vi "LCR_Readout.vi"(8 "error in (no error)":errorcluster, 11 "HP4284A in":refnum<class "HP4284A.lvclass">) -> (0 "error out":errorcluster, 1 "Resistance in Ohm":dbl, 2 "Capacitance in pF":dbl, 3 "HP4284A out":refnum<class "HP4284A.lvclass">)   [LabVIEW 2018, in "HP4284A.lvclass"]
uses:
  HP4284A.lvclass
panel:
  out "Data status":i32
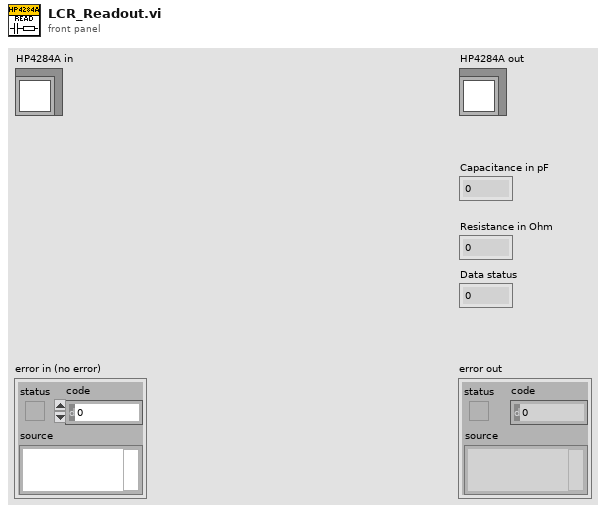
[diagram p1: front panel]
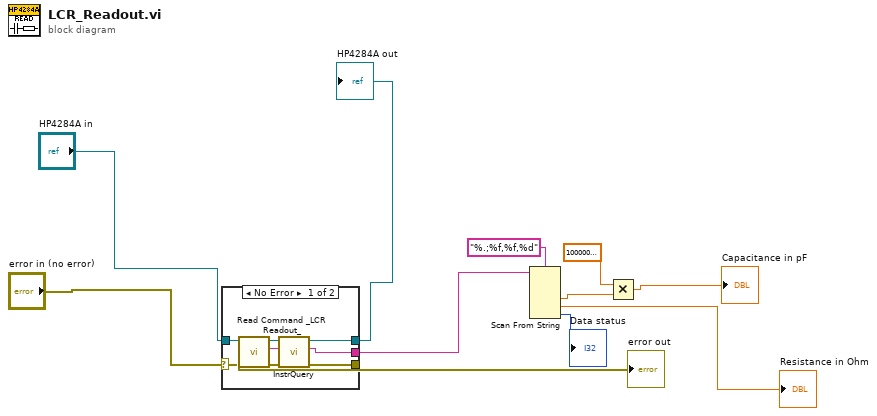
[diagram p0: block diagram]
diagram:
  n1 = case shown="No Error" "error in (no error)" {
    selector: "error in (no error)" -> [w15 w21]
    tunnel: [w14 w21] -> w11
    tunnel: [w19 w20] -> w10
    tunnel: "HP4284A in" -> [w13 w20]
    tunnel: [w12 _] -> w6
    frame No Error {
      n2 = call-dynamic "Read Command _LCR Readout_.vi"("error in (no error)"=w15, "LCRControl in"=w13) -> ("error out"=w16:errorcluster, "Command \"LCR Readout\""=w17:string, "LCRControl out"=w18:refnum<class "HP4284A.lvclass">)  [unwired: 7 in]
      n3 = call-dynamic "InstrQuery.vi"("error in (no error)"=w16, "Command string"=w17, "InstControl in"=w18) -> ("error out"=w14:errorcluster, "Instrument response"=w12:string, "InstControl out"=w19:refnum<class "HP4284A.lvclass">)  [unwired: 6 in]
    }
    frame Error {
    }
  }
  "error out" <- w11
  "HP4284A out" <- w10
  n4 = Scan From String(format string="%.;%f,%f,%d", input string=w6) -> (output 1=w5:dbl, output 2=→"Resistance in Ohm":dbl, output 3=→"Data status":i32)  [unwired: 5 in, 3 out]
  n5 = Multiply(x=1000000000000.0, y=w5) -> (x*y=→"Capacitance in pF":dbl)
